vi "7.2.Telegram_Relay_Control_with Thai Msg Response.vi"   [LabVIEW 2014]
uses:
  <vilib>/Aledyne-TSXperts/Arduino Compatible Compiler for LabVIEW/Code Generator/Arduino APIs/Digital/PinDirection.ctl
  <vilib>/Aledyne-TSXperts/Arduino Compatible Compiler for LabVIEW/addons/QwaveSys_ESP8266/QwaveSys_ESP8266.lvlib
  <vilib>/Aledyne-TSXperts/Arduino Compatible Compiler for LabVIEW/Arduino Compatible Compiler for LabVIEW.lvlib
types:
  T1 = typedef "Arduino Compatible Compiler for LabVIEW.lvlib/PinDirection.ctl" = enum16{" INPUT", "OUTPUT", " INPUT_PULLUP"}
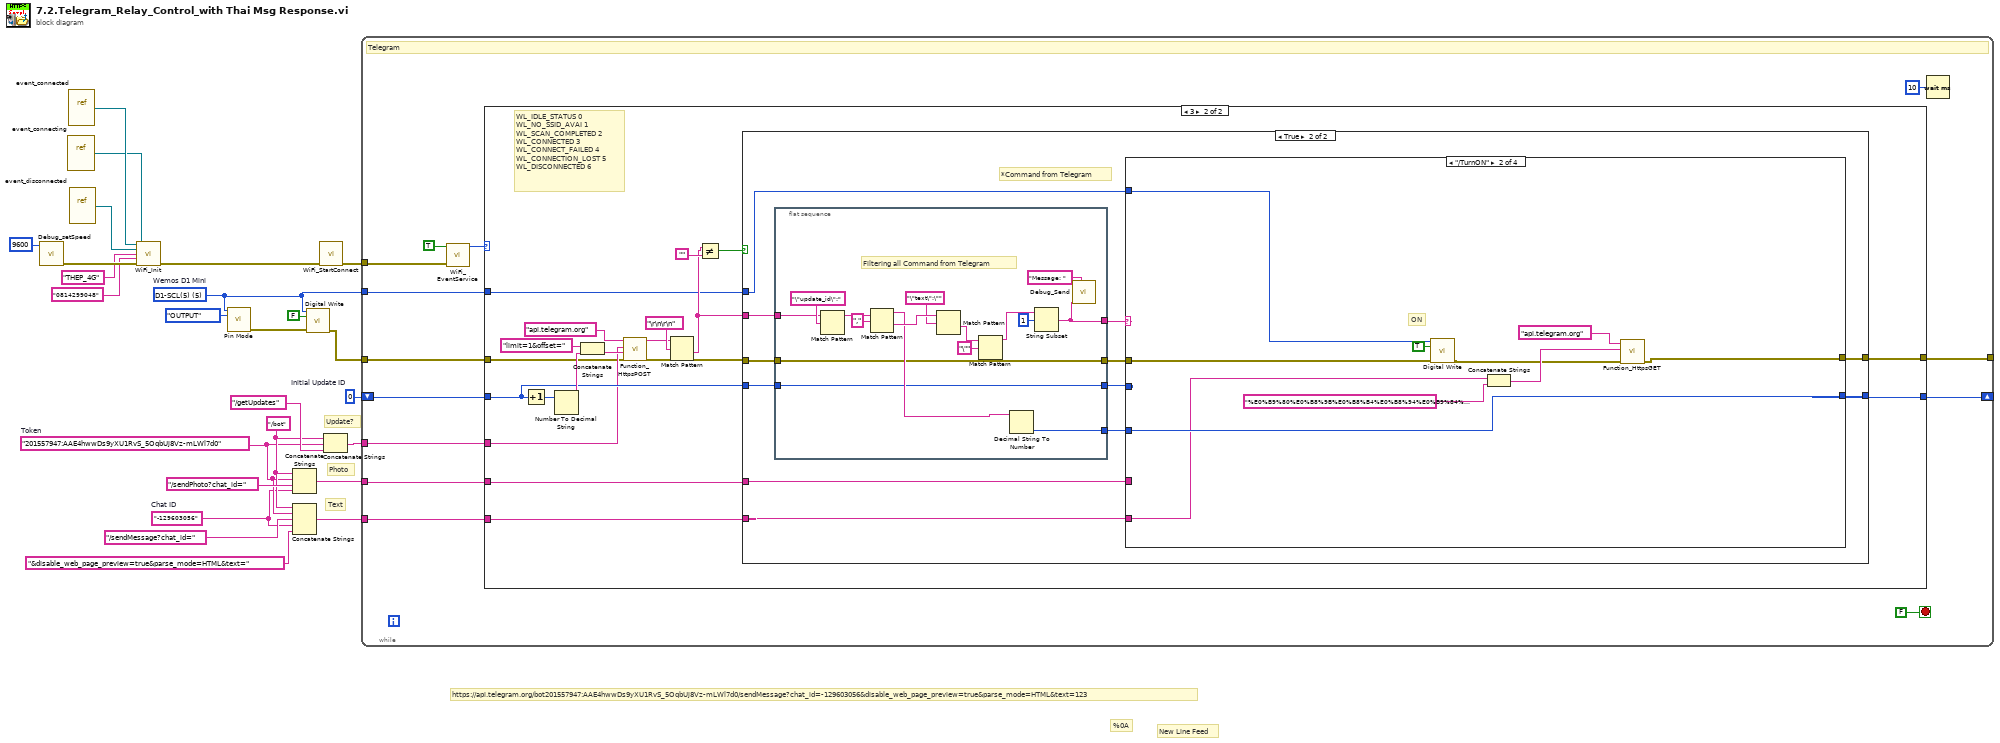
[diagram p0: block diagram]
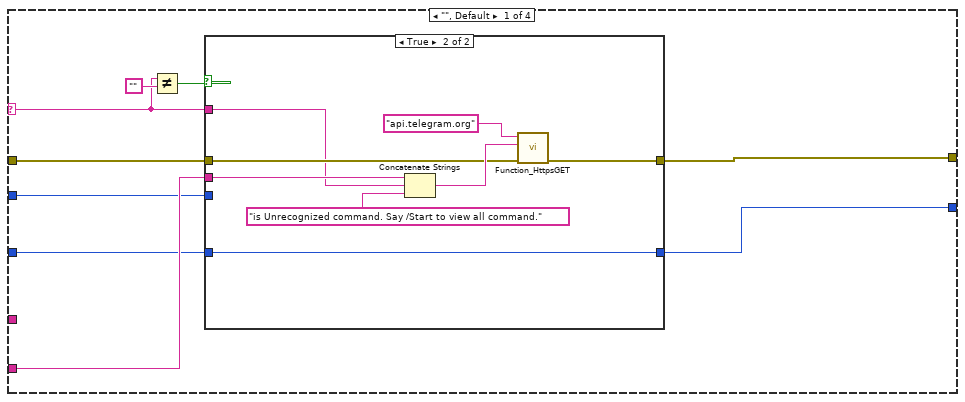
[diagram p4: hidden frame]
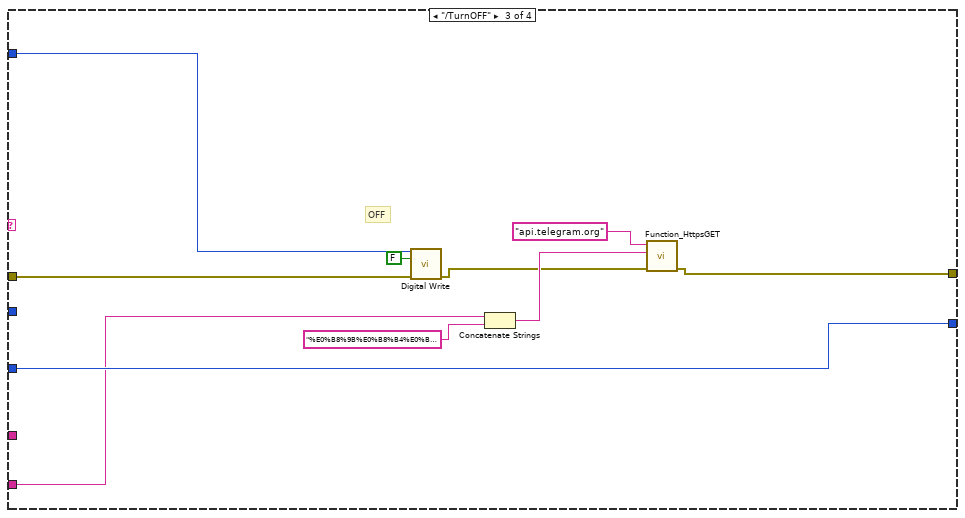
[diagram p6: hidden frame]
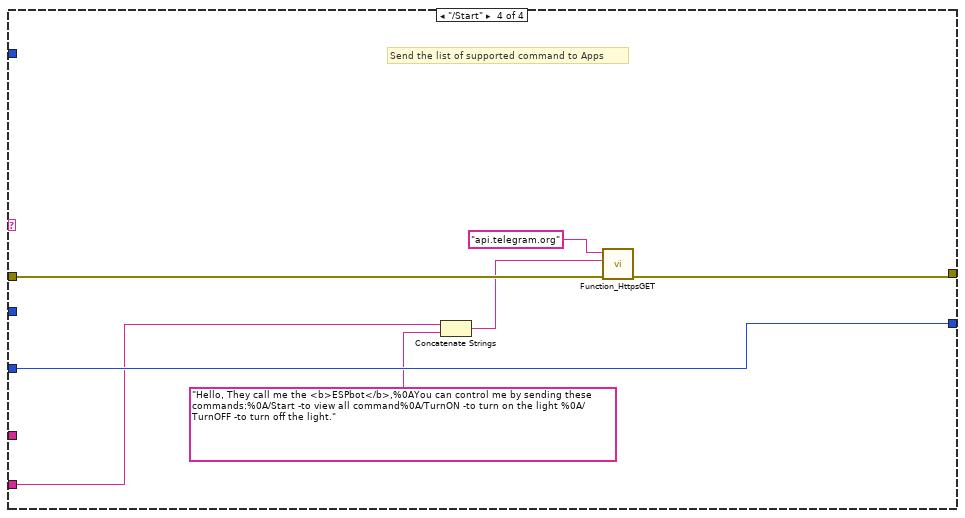
[diagram p7: hidden frame]
diagram:
  w2 = u8 5 items=["D0-(16)"=16, "D1-SCL(5)"=5, "D2-SDA(4)"=4, "D3-(0)"=0, "D4-(LED)-(2)"=2, "D5-SCK(14)"=14, "D6-MISO(12)"=12, "D7-MOSI(13)"=13, "D8-SS(15)"=15, "TX(3)"=3, "RX(1)"=1, "ADC0,(17)"=17]  # Wemos D1 Mini
  w14 = 0  # Initial Update ID
  w11 = "201557947:AAE4hwwDs9yXU1RvS_5OqbUj8Vz-mLWl7d0"  # Token
  w12 = "/bot"
  w9 = "-129603056"  # Chat ID
  # "New Line Feed"
  # "%0A"
  # "https://api.telegram.org/bot201557947:AAE4hwwDs9yXU1RvS_5OqbUj8Vz-mLWl7d0/sendMessage?chat_id=-129603056&disable_web_page_preview=true&parse_mode=HTML&text=123"
  # "Update?"
  # "Photo"
  # "Text"
  n1 = call <vilib>:"Debug_setSpeed.vi"("Speed"=u32 9600) -> ("error out"=w24:errorcluster)  [unwired: 10 in]
  n2 = vi-ref "event_connecting.vi"() -> (w20:refnum<vi>)
  n3 = vi-ref "event_connected.vi"() -> (w21:refnum<vi>)
  n4 = vi-ref "event_disconnected.vi"() -> (w19:refnum<vi>)
  n5 = call <vilib>:"WiFi_Init.vi"("connected"=w21, "connecting"=w20, "disconnected"=w19, "SSID"="THEP_4G", "PASSPHARSE"="0814299048", "error in (no error)"=w24) -> ("error out"=w1:errorcluster)  [unwired: 9 in]
  n6 = call <vilib>:"Pin Mode.vi"("pin"=w2, "direction"=PinDirection."OUTPUT") -> ("error out"=w5:errorcluster)  [unwired: 13 in]
  n7 = Concatenate Strings(w12, w11, "/sendPhoto?chat_id=", w9) -> (w13:string)
  n8 = Concatenate Strings(w12, w11, "/sendMessage?chat_id=", w9, "&disable_web_page_preview=true&parse_mode=HTML&text=") -> (w8:string)
  n9 = call <vilib>:"Digital Write.vi"("pin"=w2, "state"=FALSE, "error in (no error)"=w5) -> ("error out"=w4:errorcluster)  [unwired: 12 in]
  n10 = call <vilib>:"WiFi_StartConnect.vi"("error in (no error)"=w1) -> ("error out"=w25:errorcluster)  [unwired: 10 in]
  n11 = Concatenate Strings(w12, w11, "/getUpdates") -> (w15:string)
  n12 = while {
    tunnel: w25 -> [w37]
    tunnel: w13 -> [w32]
    tunnel: w15 -> [w33]
    shift-right: [w31] -> _
    shift-left: w14 -> [w34]
    tunnel: [w30] -> _
    tunnel: w8 -> [w28]
    tunnel: w4 -> [w27]
    tunnel: w2 -> [w26]
    stop <- FALSE stop-if-true
    # "Telegram"
    n13 = call <vilib>:"WiFi_EventService.vi"("error in (no error)"=w37, "wait for connected (True)"=TRUE) -> ("Status"=w29:u16)  [unwired: 8 in, 1 out]
    n14 = case shown="3" w29 {
      tunnel: w34 -> [w40 w46]
      tunnel: w33 -> [_ w45]
      tunnel: w32 -> [_ w53]
      tunnel: [w40 w52] -> w31
      tunnel: [w39 w51] -> w30
      tunnel: w28 -> [_ w50]
      tunnel: w27 -> [w39 w42]
      tunnel: w26 -> [_ w41]
      frame 0, Default {
      }
      frame 3 {
        # "WL_IDLE_STATUS\t0\nWL_NO_SSID_AVAI\t1\nWL_SCAN_COMPLETED\t2\nWL_CONNECTED\t3\nWL_CONNECT_FAILED\t4\nWL_CONNECTION_LOST\t5\nWL_DISCONNECTED\t6"
        n15 = Increment(x=w46) -> (x+1=w47:i32)
        n16 = Number To Decimal String(number=w47) -> (decimal integer string=w59:string)  [unwired: 1 in]
        n17 = Concatenate Strings("limit=1&offset=", w59) -> (w57:string)
        n18 = call <vilib>:"Function_HttpsPOST.vi"("error in (no error)"=w42, "DATA"=w57, "URI"=w45, "Host"="api.telegram.org") -> ("error out"=w54:errorcluster, "Results"=w48:string)  [unwired: 6 in]
        n19 = Match Pattern(string=w48, regular expression="\r\n\r\n") -> (after substring=w43:string)  [unwired: 1 in, 3 out]
        n20 = Not Equal?(x=w43, y="") -> (x != y?=w44:bool)
        n21 = case shown="True" w44 {
          tunnel: w43 -> [_ w67]
          tunnel: w54 -> [w61 w71]
          tunnel: [w61 w73] -> w51
          tunnel: w53 -> [_ w72]
          tunnel: [w60 w65] -> w52
          tunnel: w50 -> [_ w68]
          tunnel: w46 -> [w60 w64]
          tunnel: w41 -> [_ w62]
          frame False {
          }
          frame True {
            # "*Command from Telegram"
            n22 = flat-sequence {
              tunnel: [w81] -> w66
              tunnel: w71 -> [w80]
              tunnel: [w80] -> w70
              tunnel: [w77] -> w69
              tunnel: w67 -> [w76]
              tunnel: [w74] -> w63
              tunnel: w64 -> [w74]
              frame #0 {
                # "Filtering all Command from Telegram"
                n23 = Match Pattern(string=w76, regular expression="\"update_id\":") -> (after substring=w84:string)  [unwired: 1 in, 3 out]
                n24 = Match Pattern(string=w84, regular expression=",") -> (before substring=w82:string, after substring=w89:string)  [unwired: 1 in, 2 out]
                n25 = Match Pattern(string=w89, regular expression="\"text\":\"") -> (after substring=w87:string)  [unwired: 1 in, 3 out]
                n26 = Match Pattern(string=w87, regular expression="\"") -> (before substring=w78:string)  [unwired: 1 in, 3 out]
                n27 = Decimal String To Number(string=w82) -> (number=w81:i32)  [unwired: 2 in, 1 out]
                n28 = String Subset(string=w78, offset (0)=1) -> (substring=w77:string)  [unwired: 1 in]
                n29 = call <vilib>:"Debug_Send.vi"("Name"="Message: ", "DATA"=w77) -> ()  [unwired: 10 in]
              }
            }
            n30 = case shown="\"/TurnON\"" w69 {
              selector: w69 -> [w90 _ _ _]
              tunnel: w70 -> [w98 w118 w128 w134]
              tunnel: w72 -> [_ _ _ _]
              tunnel: [w97 w109 w120 w133] -> w73
              tunnel: w68 -> [w96 w111 w122 w130]
              tunnel: w66 -> [w93 w115 w125 w132]
              tunnel: [w92 w115 w125 w132] -> w65
              tunnel: w63 -> [w91 _ _ _]
              tunnel: w62 -> [_ w117 w127 _]
              frame "", Default {
                n31 = Not Equal?(x=w90, y="" ("Empty String Constant")) -> (x != y?=w94:bool)
                n32 = case shown="True" w94 {
                  tunnel: w98 -> [w100 w106]
                  tunnel: [w100 w105] -> w97
                  tunnel: w96 -> [_ w104]
                  tunnel: w90 -> [_ w103]
                  tunnel: w93 -> [_ w101]
                  tunnel: [w99 w101] -> w92
                  tunnel: w91 -> [w99 _]
                  frame False {
                  }
                  frame True {
                    n33 = Concatenate Strings(w104, w103, "is Unrecognized command. Say /Start to view all command." ("string")) -> (w107:string)
                    n34 = call <vilib>:"Function_HttpsGET.vi"("error in (no error)"=w106, "URI"=w107, "Host"="api.telegram.org") -> ("error out"=w105:errorcluster)  [unwired: 7 in, 1 out]
                  }
                }
              }
              frame "/TurnON" {
                # "ON"
                n35 = call <vilib>:"Digital Write.vi"("pin"=w117, "state"=TRUE, "error in (no error)"=w118) -> ("error out"=w112:errorcluster)  [unwired: 12 in]
                n36 = Concatenate Strings(w111, "%E0%B9%80%E0%B8%9B%E0%B8%B4%E0%B8%94%E0%B9%84%E0%B8%9F%E0%B9%83%E0%B8%AB%E0%B9%89%E0%B9%81%E0%B8%A5%E0%B9%89%E0%B8%A7%E0%B8%84%E0%B9%88%E0%B8%B0...") -> (w113:string)
                n37 = call <vilib>:"Function_HttpsGET.vi"("error in (no error)"=w112, "URI"=w113, "Host"="api.telegram.org") -> ("error out"=w109:errorcluster)  [unwired: 7 in, 1 out]
              }
              frame "/TurnOFF" {
                # "OFF"
                n38 = call <vilib>:"Digital Write.vi"("pin"=w127, "state"=FALSE, "error in (no error)"=w128) -> ("error out"=w121:errorcluster)  [unwired: 12 in]
                n39 = Concatenate Strings(w122, "%E0%B8%9B%E0%B8%B4%E0%B8%94%E0%B9%84%E0%B8%9F%E0%B9%81%E0%B8%A5%E0%B9%89%E0%B8%A7%E0%B8%84%E0%B9%88%E0%B8%B0%21") -> (w123:string)
                n40 = call <vilib>:"Function_HttpsGET.vi"("error in (no error)"=w121, "URI"=w123, "Host"="api.telegram.org") -> ("error out"=w120:errorcluster)  [unwired: 7 in, 1 out]
              }
              frame "/Start" {
                # "Send the list of supported command to Apps"
                n41 = Concatenate Strings(w130, "Hello, They call me the <b>ESPbot</b>,%0AYou can control me by sending these commands:%0A/Start -to view all command%0A/TurnON -to turn on the light %0A/TurnOFF -to turn off the light.") -> (w131:string)
                n42 = call <vilib>:"Function_HttpsGET.vi"("error in (no error)"=w134, "URI"=w131, "Host"="api.telegram.org") -> ("error out"=w133:errorcluster)  [unwired: 7 in, 1 out]
              }
            }
          }
        }
      }
    }
    n43 = Wait (ms)(milliseconds to wait=u32 10) -> ()  [unwired: 1 out]
  }
